vi "ConsistancyCheck.vi"(2 "Input 2":dbl[](array[numeric]), 3 "Input 1":dbl[](array[numeric])) -> (0 "Slope Difference":dbl, 1 "Difference":dbl)   [LabVIEW 2017]
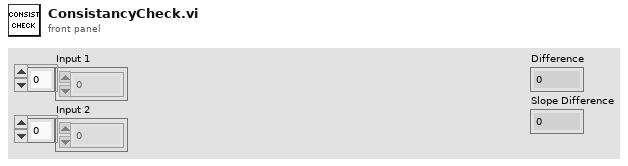
[diagram p1: front panel]
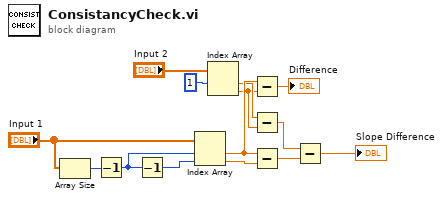
[diagram p0: block diagram]
diagram:
  n1 = Array Size(array="Input 1") -> (size(s)=w13:i32)
  n2 = Decrement(x=w13) -> (x-1=w12:i32)
  n3 = Decrement(x=w12) -> (x-1=w2:i32)
  n4 = Index Array(array="Input 1", index #1=w12, index #2=w2) -> (element #1=w8:dbl, element #2=w1:dbl)
  n5 = Index Array(array="Input 2", index #1=1 ("index")) -> (element #1=w7:dbl, element #2=w3:dbl)  [unwired: 1 in]
  n6 = Subtract(x=w8, y=w3) -> (x-y=→"Difference":dbl)
  n7 = Subtract(x=w7, y=w3) -> (x-y=w4:dbl)
  n8 = Subtract(x=w8, y=w1) -> (x-y=w5:dbl)
  n9 = Subtract(x=w4, y=w5) -> (x-y=→"Slope Difference":dbl)
